vi "OneVector.vi"() -> ()   [LabVIEW 2022 SP3, in "Vector2.lvclass"]
uses:
  Vector2.lvclass
  Vector2.lvclass/Vector2.ctl
panel:
  out "One Vector":refnum<class "Vector2.lvclass">
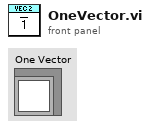
[diagram p1: front panel]
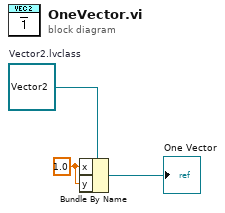
[diagram p0: block diagram]
diagram:
  w1 = 1.0 ("x")
  w2 = refnum<class "Vector2.lvclass"> refnum  # Vector2.lvclass
  n1 = Bundle By Name(cluster=w2, "x"=w1, "y"=w1) -> (→"One Vector":refnum<class "Vector2.lvclass">)
